vi "Button Toggle (Sub).vi"(11 "Buttons":bool[](array[boolean])) -> (1 "toggle on press and on release 3":bool, 2 "toggle on relase 3":bool, 3 "toggle on press 3":bool)   [LabVIEW 2020]
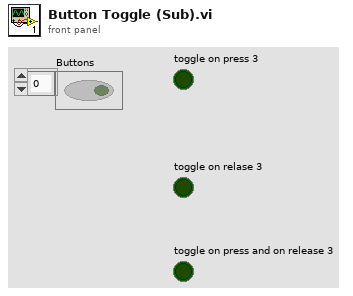
[diagram p1: front panel]
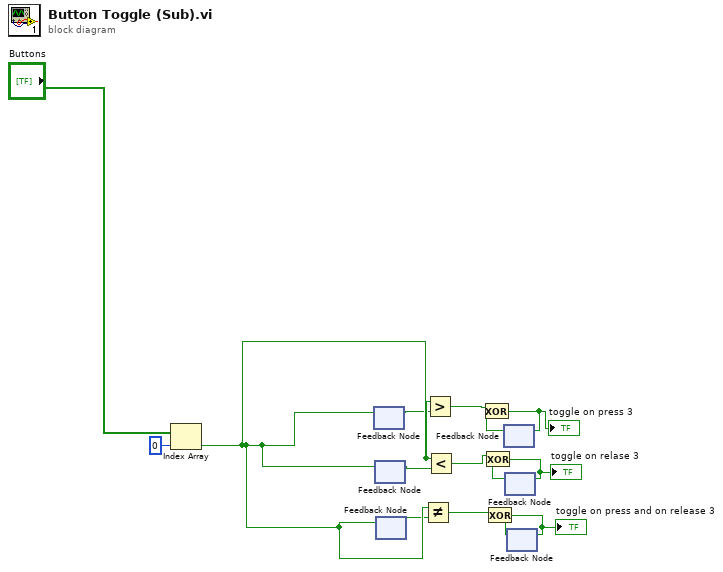
[diagram p0: block diagram]
diagram:
  n1 = Index Array(array="Buttons", index=0) -> (element=w14:bool)
  n2 = feedback #1() -> (w1:bool)  [unwired: 1 in]
  n3 = feedback-in #1(w14) -> ()
  n4 = feedback #2() -> (w12:bool)  [unwired: 1 in]
  n5 = feedback-in #2(w14) -> ()
  n6 = feedback #3() -> (w7:bool)  [unwired: 1 in]
  n7 = feedback-in #3(w14) -> ()
  n8 = Not Equal?(x=w14, y=w7) -> (x != y?=w8:bool)
  n9 = Greater?(x=w14, y=w1) -> (0:w2:bool)
  n10 = Less?(x=w14, y=w12) -> (x < y?=w11:bool)
  n11 = feedback #4() -> (w3:bool)  [unwired: 1 in]
  n12 = Exclusive Or(1:w3, 2:w2) -> (0:w4:bool)
  "toggle on press 3" <- w4
  n13 = feedback-in #4(w4) -> ()
  n14 = feedback #5() -> (w10:bool)  [unwired: 1 in]
  n15 = Exclusive Or(1:w10, 2:w11) -> (0:w5:bool)
  "toggle on relase 3" <- w5
  n16 = feedback-in #5(w5) -> ()
  n17 = feedback #6() -> (w9:bool)  [unwired: 1 in]
  n18 = Exclusive Or(1:w9, 2:w8) -> (0:w6:bool)
  "toggle on press and on release 3" <- w6
  n19 = feedback-in #6(w6) -> ()
